vi "Collect force curve segement metadata.vi"(0 "reference in":refnum<class "metadata.lvclass">, 5 "error in (no error)":errorcluster) -> (10 "Segment Header":string, 14 "reference out":refnum<class "metadata.lvclass">, 15 "List property names":string, 16 "Metadata":T1, 19 "error out":errorcluster)   [LabVIEW 2019, in "metadata.lvclass"]
uses:
  metadata.lvclass
  Metadata output --cluster.ctl
  Force curve segment type--combobox.ctl
panel:
  out "Fcurve segment.nb":u8
  out "Property Names":string[](array[string])
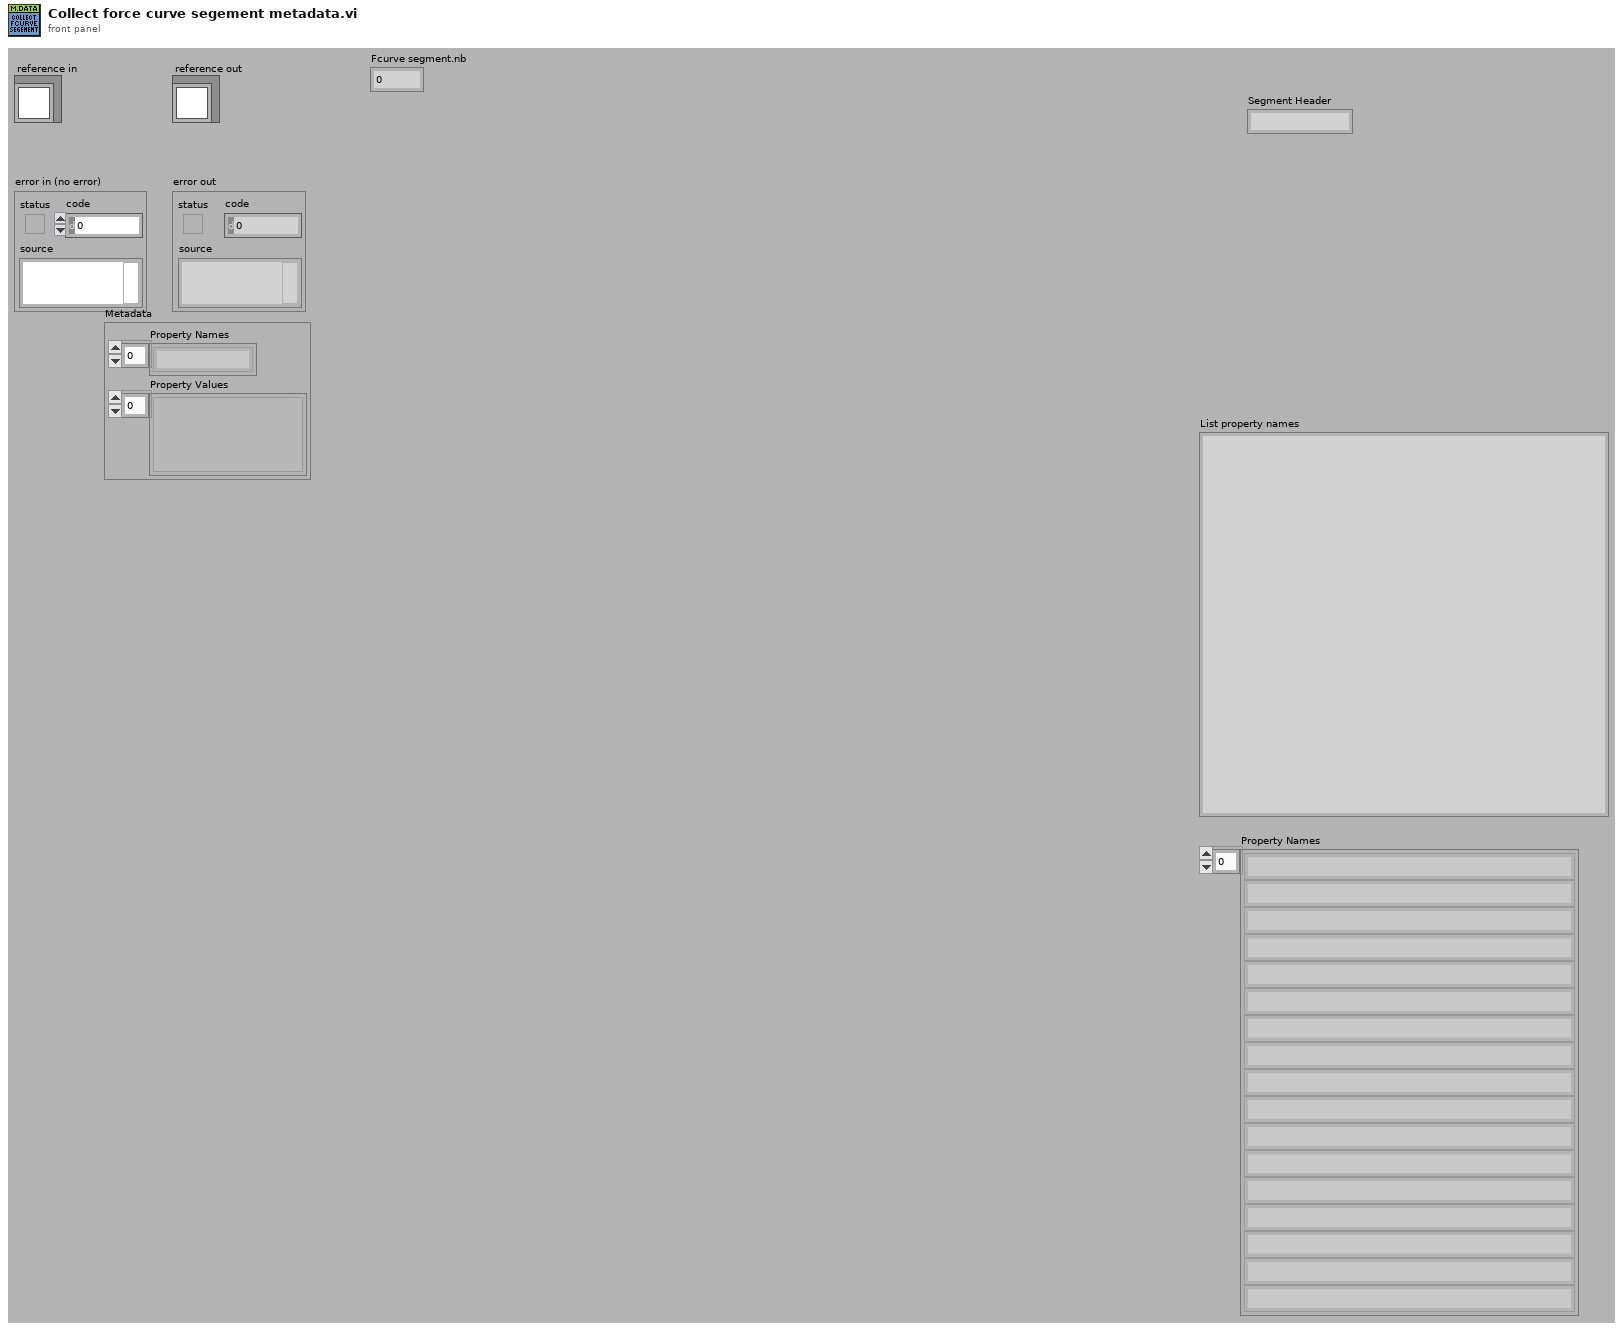
[diagram p1: front panel]
types:
  T1 = typedef "metadata.lvclass/Metadata output --cluster.ctl" = cluster{"Property Names":string[], "Property Values":variant[]}
  T2 = typedef "metadata.lvclass/Force curve segment type--combobox.ctl" = string
  T3 = typedef "metadata.lvclass/ObjectAttributes.ctl" = cluster{"MyAttribute":dbl, "System Control":T4, "file info":T5, "Sample info":T6, "Cantilever info":T7, "XYZ piezos":T8, "Mapping":T9, "Fcurve segment":T10[], "Fast fpga segment":T12, "Chirp":T13, "precision (6)":i16, "width (-)":i16, "Metadata":T1, "config filepath":path, "Section names []":string[], "Property names []":string[], "nb elements":u16}
  T4 = typedef "metadata.lvclass/System control parameters.ctl" = cluster{"FPGA SW version":string, "TDMS file version":string, "Instrument":string, "Instrument model":string, "Instrument scanner":string, "Instrument clockrate (Mhz)":string, "Instrument tick time (us)":string}
  T5 = typedef "metadata.lvclass/File info parameters.ctl" = cluster{"Time Stamp":timestamp, "Filename":string, "Filepath":path, "User":string, "Experiment_name":string, "Curve_id":string, "number_segments":u8, "number_consecutive_scans":u32}
  T6 = typedef "metadata.lvclass/Sample info parameters.ctl" = cluster{"Sample name":string, "Sample species":string}
  T7 = typedef "metadata.lvclass/Cantilever info parameters.ctl" = cluster{"spring constant calib method":string, "invOLS calib method":string, "thermal calib deflection channel":string, "model":string, "shape":string, "tip geometry":string, "Laser sum (V)":dbl, "Laser power (mA)":dbl, "invOLS_(nm/V)":dbl, "spring constant nominal (N/m)":dbl, "spring constant calib (N/m)":dbl, "resosnance frequency air calib (Hz)":dbl, "resosnance frequency calib (Hz)":dbl, "quality factor":dbl, "Acoefficident_GCI_(nN.s^1.3/m)":dbl, "half angle (deg)":dbl, "tip radius (m)":dbl, "tip height (m)":dbl, "system mount angle (deg)":dbl}
  T8 = typedef "metadata.lvclass/XYZ piezos parameters.ctl" = cluster{"X stage piezo sensitivity (nm/V)":dbl, "X stage piezo gain":dbl, "X velocity (V/tick)":dbl, "X closed loop":bool, "Y stage piezo sensitivity (nm/V)":dbl, "Y stage piezo gain":dbl, "Y velocity (V/tick)":dbl, "Y closed loop":bool, "Z stage piezo sensitivity (nm/V)":dbl, "Z stage piezo gain":dbl, "Z closed loop":bool, "X position (V)":dbl, "Y position (V)":dbl}
  T9 = typedef "metadata.lvclass/Mapping parameters.ctl" = cluster{"Mapping":bool, "index":u16, "position row":u16, "position column":u16, "next position row":i16, "next position column":i16, "X initial position (V)":dbl, "Y initial position (V)":dbl, "X step size (V)":dbl, "Y step size (V)":dbl}
  T10 = typedef "metadata.lvclass/Fcurve segment.ctl" = cluster{"type":T11, "fast_fpga_trigger":bool, "nb":u8, "duration (ticks)":i64, "nb points":i32, "sampling rate (S/s)":u32, "Zpiezo control out":string, "initial deflection (V)":dbl, "relative setpoint":bool, "setpoint on":bool, "setpoint (V)":dbl, "setpoint trigger channel":string, "velocity (V/tick)":dbl, "Z position setpoint trigger (V)":dbl, "Z retract length (V)":dbl, "dec factor":u32}
  T11 = typedef "metadata.lvclass/Segment type--combobox.ctl" = string
  T12 = typedef "metadata.lvclass/fast fpga segment parameters.ctl" = cluster{"Fast start time trigger":timestamp, "nb_points":u32, "sampling_rate_(S/s)":u32, "duration_(ticks)":u32}
  T13 = typedef "metadata.lvclass/Chirp added parameters.ctl" = cluster{"f start (Hz)":dbl, "f end (Hz)":dbl, "Sweep type":string}
  T14 = cluster{"Property Names":string[], "Property Values":variant[]}
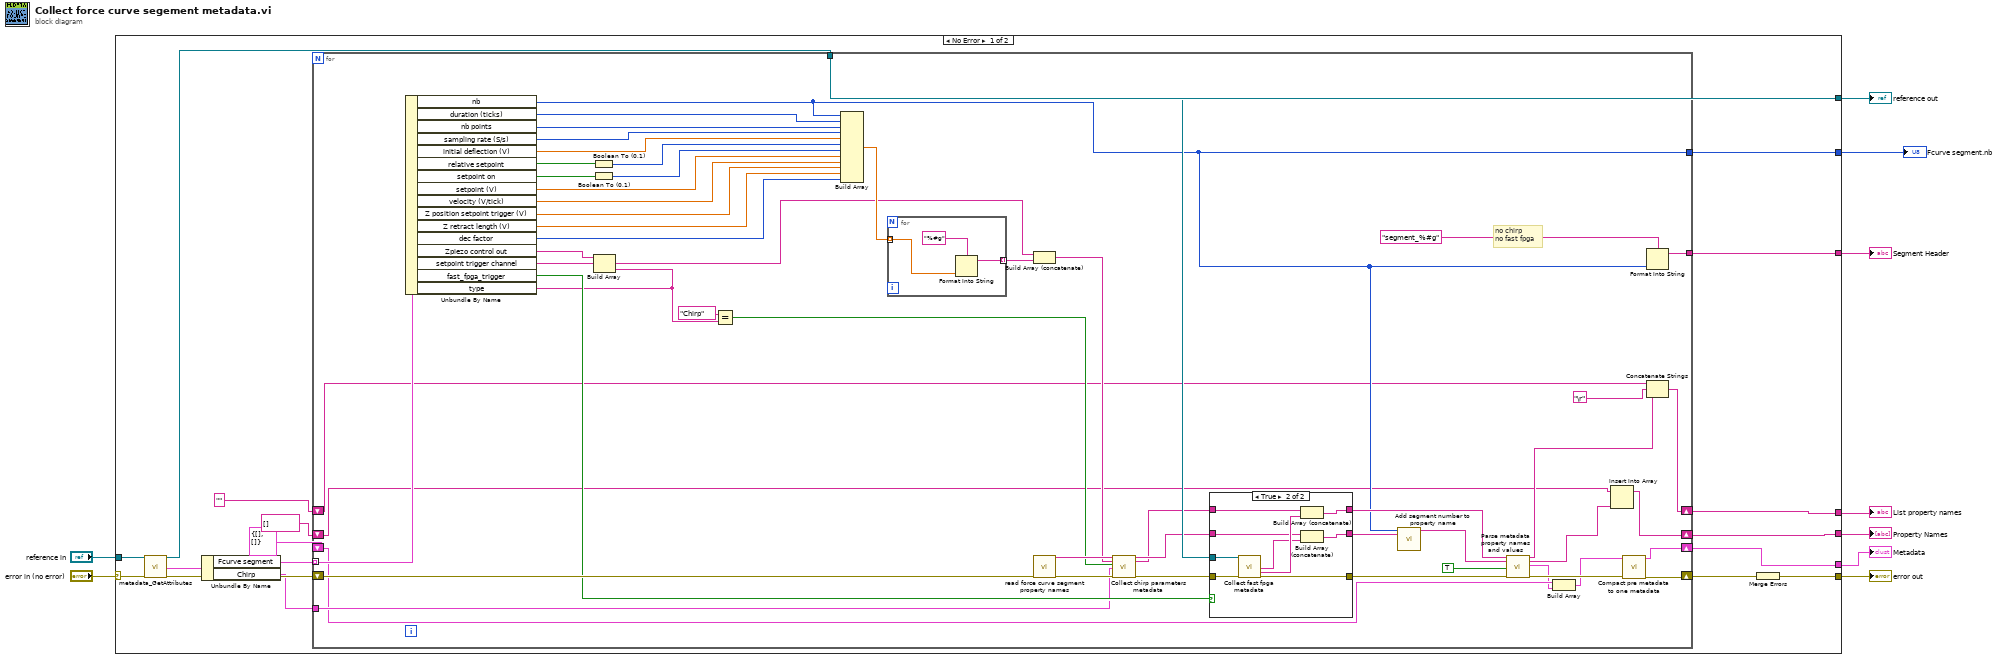
[diagram p0: block diagram]
diagram:
  n1 = case shown="No Error" "error in (no error)" {
    selector: "error in (no error)" -> [w24 w96]
    tunnel: [w26 w96] -> w8
    tunnel: [w18 w95] -> w6
    tunnel: "reference in" -> [w25 w95]
    tunnel: [w22 _] -> w5
    tunnel: [w21 _] -> w3
    tunnel: [w20 _] -> w4
    tunnel: [w17 _] -> w2
    tunnel: [w16 _] -> w1
    frame No Error {
      n2 = call "metadata_GetAttributes.vi"("reference in"=w25, "error in (no error)"=w24) -> ("reference out"=w18:refnum<class "metadata.lvclass">, "attributes"=w15:T3, "error out"=w19:errorcluster)  [unwired: 14 in, 1 out]
      n3 = Unbundle By Name(w15) -> ("Fcurve segment"=w14:T10[], "Chirp"=w13:T13)
      n4 = for {
        tunnel: w18 -> [w53]
        tunnel: [w44] -> w17
        tunnel: [w42] -> w16
        shift-right: [w31] -> w23
        shift-left: w19 -> [w77]
        tunnel: w14 -> [w41] mode=indexing
        tunnel: w13 -> [w40]
        shift-right: [w36] -> w20
        shift-left: "" ("Param list") -> [w39]
        shift-right: [w33] -> w22
        shift-left: string[] [] -> [w34]
        shift-right: [w27] -> w21
        shift-left: T1 {"Property Names"=[], "Property Values"=[]} ("output cluster") -> [w30]
        # "no chirp\nno fast fpga"
        n5 = Unbundle By Name(w41) -> ("nb"=w42:u8, "duration (ticks)"=w76:i64, "nb points"=w75:i32, "sampling rate (S/s)"=w74:u32, "initial deflection (V)"=w73:dbl, "relative setpoint"=w72:bool, "setpoint on"=w71:bool, "setpoint (V)"=w68:dbl, "velocity (V/tick)"=w67:dbl, "Z position setpoint trigger (V)"=w66:dbl, "Z retract length (V)"=w65:dbl, "dec factor"=w64:u32, "Zpiezo control out"=w62:string, "setpoint trigger channel"=w61:string, "fast_fpga_trigger"=w46:bool, "type"=w43:T11)
        n6 = Boolean To (0,1)(Boolean=w72) -> (0, 1=w70:i16)
        n7 = Boolean To (0,1)(Boolean=w71) -> (0, 1=w69:i16)
        n8 = Build Array(w62, w61, w43) -> (w60:T11[])
        n9 = Equal?(x=T2 "Chirp", y=w43) -> (x = y?=w47:bool)
        n10 = Build Array(w42, w76, w75, w74, w73, w70, w69, w68, w67, w66, w65, w64) -> (w63:dbl[])
        n11 = for {
          tunnel: [w93] -> w79 mode=indexing
          tunnel: w63 -> [w92] mode=indexing
          n12 = Format Into String(format string="%#g", w92) -> (resulting string=w93:string)  [unwired: 2 in, 1 out]
        }
        n13 = Build Array (concatenate)(w60, w79) -> (w56:T11[])
        n14 = call "read force curve segment property names.vi"("error in (no error)"=w77) -> ("Fcurve Seg"=w59:string[], "error out"=w57:errorcluster)  [unwired: 17 in]
        n15 = call "Collect chirp parameters metadata.vi"("Property Names in"=w59, "Property Values in"=w56, "Chirp?"=w47, "Chirp"=w40, "error in (no error)"=w57) -> ("Property names out"=w52:string[], "Property values out"=w51:string[], "error out"=w55:errorcluster)  [unwired: 12 in]
        n16 = case shown="True" w46 {
          tunnel: w55 -> [w82 w91]
          tunnel: [w82 w90] -> w54
          tunnel: w53 -> [_ w89]
          tunnel: w52 -> [w80 w86]
          tunnel: w51 -> [w81 w88]
          tunnel: [w80 w84] -> w49
          tunnel: [w81 w83] -> w50
          frame False {
          }
          frame True {
            n17 = call-dynamic "Collect fast fpga metadata.vi"("reference in"=w89, "error in (no error)"=w91) -> ("Property Names"=w85:string[], "Property values"=w87:string[], "error out"=w90:errorcluster)  [unwired: 13 in, 2 out]
            n18 = Build Array (concatenate)(w88, w87) -> (w83:string[])
            n19 = Build Array (concatenate)(w86, w85) -> (w84:string[])
          }
        }
        n20 = call "Add segment number to property name.vi"("Fcurve segment.nb"=w42, "Property Name"=w49) -> ("Segment_#_propertyName"=w48:string[])  [unwired: 17 in]
        n21 = call "Parse metadata property names and values.vi"("Data intput []"=w50, "property names []"=w48, "List param"=TRUE, "error in (no error)"=w54) -> ("Param list"=w37:string, "Array"=w35:string[], "output cluster"=w29:T1, "error out"=w32:errorcluster)  [unwired: 12 in]
        n22 = Build Array(w30, w29) -> (w28:T1[])
        n23 = Insert Into Array(array=w34, new element=w35) -> (w33:string[])  [unwired: 1 in]
        n24 = call "Compact pre metadata to one metadata.vi"("appended array"=w28, "error in (no error)"=w32) -> ("Metadata"=w27:T14, "error out"=w31:errorcluster)  [unwired: 16 in]
        n25 = Format Into String(format string="segment_%#g", w42) -> (resulting string=w44:string)  [unwired: 2 in, 1 out]
        n26 = Concatenate Strings(w39, "\r", w37) -> (w36:string)
      }
      n27 = Merge Errors(w23) -> (w26:errorcluster)
    }
    frame Error {
    }
  }
  "error out" <- w8
  "reference out" <- w6
  "Property Names" <- w5
  "List property names" <- w4
  "Metadata" <- w3
  "Segment Header" <- w2
  "Fcurve segment.nb" <- w1
